vi "HTTP Method.vi"(0 "REST Client_NET in":refnum<class "REST Client_NET.lvclass">, 1 "Method":T2, 5 "Path":string, 7 "Request body":string, 9 "Multipart Post data":T1[](array[typedef]), 11 "error in (no error)":errorcluster, 12 "request specific headers":T3[](array[typedef]), 13 "timeout (0 = Use Default)":i32) -> (2 "ReasonPhrase":string, 3 "StatusCode":i32, 4 "REST Client_NET out":refnum<class "REST Client_NET.lvclass">, 6 "Response Headers out":refnum<class "Response Headers.lvclass">, 8 "Response":string, 15 "error out":errorcluster)   [LabVIEW 2018, in "REST Client_NET.lvlib" / "REST Client_NET.lvclass"]
doc: "<b> </b> <b> </b>\nHttpClient_NET\nJustin Young - Viviota\nCopyright (c) 2021\nLicense: BSD"
uses:
  REST Client_NET.lvclass
  C:/Program Files (x86)/National Instruments/LabVIEW 2018/vi.lib/addons/_JKI.lib/REST Client/classes/REST Client/REST Client.lvclass
  <vilib>/addons/_JKI.lib/REST Client/classes/REST Client/HTTP Header.ctl
  <vilib>/addons/_JKI.lib/REST Client/classes/REST Client/HTTP Methods.ctl
  <vilib>/httpClient/MultipartData.ctl
  <vilib>/addons/_JKI.lib/REST Client/classes/Response Headers/Response Headers.lvclass
  Rest Client Headers_NET/REST Client Headers_NET.lvclass
  C:/Program Files (x86)/National Instruments/LabVIEW 2018/vi.lib/addons/_JKI.lib/REST Client/classes/Response Headers/Response Headers.lvclass
  <vilib>/addons/_JKI.lib/REST Client/classes/REST Client/REST Client.lvclass
  <vilib>/httpClient/LabVIEWHTTPClient.lvlib
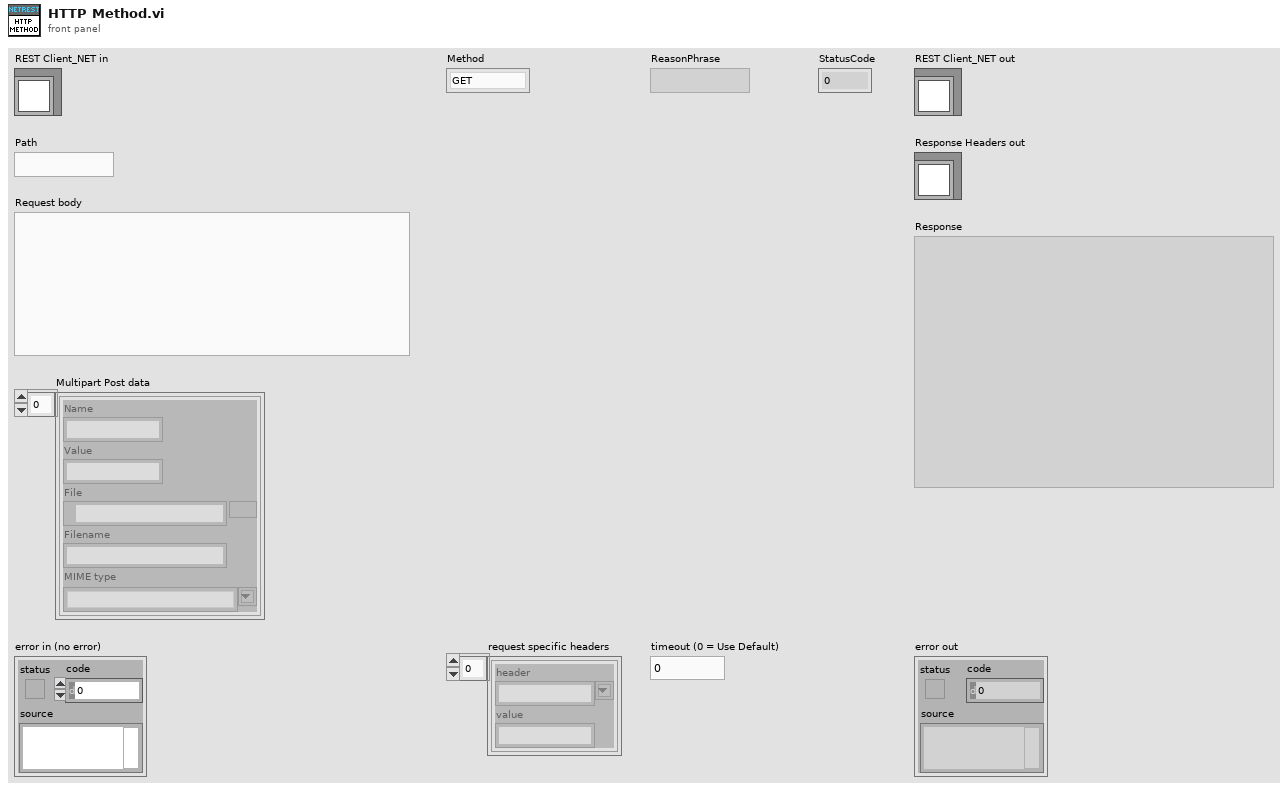
[diagram p1: front panel]
types:
  T1 = typedef "LabVIEWHTTPClient.lvlib/MultipartData.ctl" = cluster{"Name":string, "Value":string, "File":path, "Filename":string, "MIME type":string}
  T2 = typedef "REST Client.lvlib/REST Client.lvclass/HTTP Methods.ctl" = enum16{"GET", "HEAD", "POST", "PUT", "DELETE"}
  T3 = typedef "REST Client.lvlib/REST Client.lvclass/HTTP Header.ctl" = cluster{"header":string, "value":string}
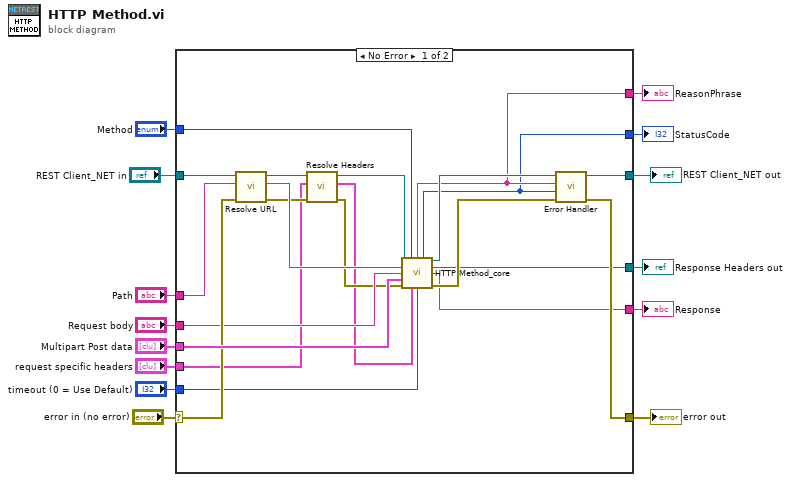
[diagram p0: block diagram]
diagram:
  n1 = case shown="No Error" "error in (no error)" {
    selector: "error in (no error)" -> [w32 w38]
    tunnel: [w30 w38] -> w10
    tunnel: [w36 w37] -> w11
    tunnel: "REST Client_NET in" -> [w33 w37]
    tunnel: "Method" -> [w25 _]
    tunnel: "Path" -> [w35 _]
    tunnel: "Request body" -> [w28 _]
    tunnel: "request specific headers" -> [w16 _]
    tunnel: "Multipart Post data" -> [w34 _]
    tunnel: "timeout (0 = Use Default)" -> [w26 _]
    tunnel: [w24 _] -> w4
    tunnel: [w23 _] -> w3
    tunnel: [w22 _] -> w2
    tunnel: [w21 _] -> w1
    frame No Error {
      n2 = call <vilib>:"Resolve URL.vi"("error in (no error)"=w32, "Path"=w35, "REST Client in"=w33) -> ("error out"=w18:errorcluster, "Resolved URL"=w29:string, "REST Client out"=w20:refnum<class "REST Client_NET.lvclass">)  [unwired: 6 in]
      n3 = call <vilib>:"Resolve Headers.vi"("error in (no error)"=w18, "headers in"=w16, "REST Client in"=w20) -> ("error out"=w17:errorcluster, "headers out"=w15:T3[], "REST Client out"=w19:refnum<class "REST Client_NET.lvclass">)  [unwired: 6 in]
      n4 = call "HTTP Method_core.vi"("REST Client_NET in"=w19, "Method"=w25, "Resolved URL"=w29, "Request body"=w28, "Multipart Post data"=w34, "error in (no error)"=w17, "request specific headers"=w15, "timeout (0 = Use Default)"=w26) -> ("ReasonPhrase"=w22:string, "StatusCode"=w21:i32, "REST Client_NET out"=w27:refnum<class "REST Client_NET.lvclass">, "REST Client Headers_NET out"=w23:refnum<class "REST Client Headers_NET.lvclass">, "Response"=w24:string, "error out"=w31:errorcluster)  [unwired: 2 in]
      n5 = call-dynamic "Error Handler.vi"("error in (no error)"=w31, "Status Code"=w21, "Status String"=w22, "REST Client in"=w27) -> ("error out"=w30:errorcluster, "REST Client out"=w36:refnum<class "REST Client_NET.lvclass">)  [unwired: 6 in]
    }
    frame Error {
    }
  }
  "error out" <- w10
  "REST Client_NET out" <- w11
  "Response Headers out" <- w3
  "ReasonPhrase" <- w2
  "StatusCode" <- w1
  "Response" <- w4
